vi "Point in Polygon (Scalar).vi"(6 "tolerance":dbl=1e-09, 8 "Polygon Y":dbl[](array[numeric]), 9 "Polygon X":dbl[](array[numeric]), 10 "y":dbl, 11 "x":dbl) -> (0 "error":i32, 3 "position":T1 items=["Inside", "On Boundary", "Outside"])   [LabVIEW 2017, in "NI_AAL_Geometry.lvlib"]
doc: "Verifies whether a point is inside a polygon."
uses:
  <vilib>/Analysis/NI_AAL_Geometry.lvlib
  <vilib>/Analysis/geometry.llb/Point in Polygon Position.ctl
panel:
  # "Point in Polygon (Scalar)"
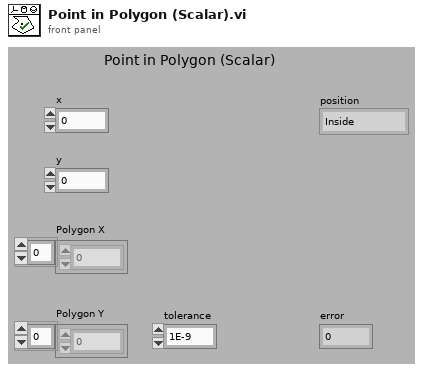
[diagram p1: front panel]
types:
  T1 = typedef "NI_AAL_Geometry.lvlib/Point in Polygon Position.ctl" = u16
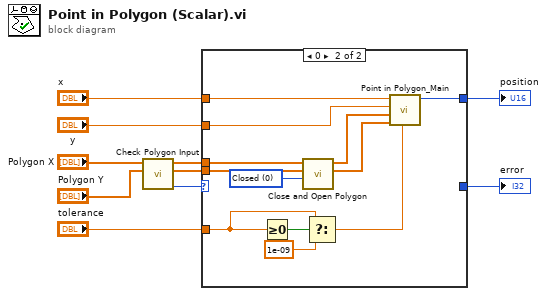
[diagram p0: block diagram]
diagram:
  n1 = call <vilib>:"Check Polygon Input.vi"("Y In"="Polygon Y", "X In"="Polygon X") -> ("error"=w10:i32, "Y Out"=w4:dbl[], "X Out"=w5:dbl[])  [unwired: 7 in]
  n2 = case shown="0" w10 {
    selector: w10 -> [w11 _]
    tunnel: w5 -> [_ w22]
    tunnel: [w11 _] -> w1
    tunnel: "x" -> [_ w18]
    tunnel: "y" -> [_ w17]
    tunnel: [_ w16] -> w2
    tunnel: "tolerance" -> [_ w14]
    tunnel: w4 -> [_ w21]
    frame -1, Default {
    }
    frame 0 {
      w23 = u16 0 items=["Closed", "Open"] ("type")
      n3 = Greater Or Equal To 0?(x=w14) -> (x >= 0?=w15:bool)
      n4 = call <vilib>:"Close and Open Polygon.vi"("type"=w23, "Y In"=w21, "X In"=w22) -> ("Y Out"=w20:dbl[], "X Out"=w19:dbl[])  [unwired: 7 in]
      n5 = Select(t=w14, s=w15, f=1e-09) -> (s? t:f=w12:dbl)
      n6 = call <vilib>:"Point in Polygon_Main.vi"("tolerance"=w12, "Polygon Y"=w20, "Polygon X"=w19, "y"=w17, "x"=w18) -> ("position"=w16:T1)  [unwired: 6 in]
    }
  }
  "error" <- w1
  "position" <- w2
